vi "TestReadWrite.vi"() -> ()   [LabVIEW 2017, in "JKI Simple Localization.lvlib"]
uses:
  API/JKI Simple Localization.lvlib
panel:
  out "error out":errorcluster
  in  "Dictionary File Path":path
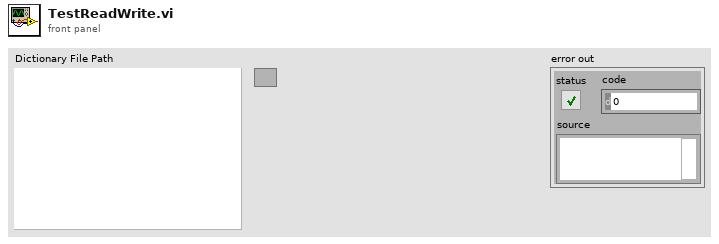
[diagram p1: front panel]
types:
  T1 = typedef "JKI Simple Localization.lvlib/Dictionary--Cluster.ctl" = cluster{"Languages":string[], "Fonts":T2[], "Phrase Dictionary":T3[]}
  T2 = typedef "JKI Simple Localization.lvlib/FontCluster.ctl" = cluster{"Language":string, "Name":string, "Color":u32}
  T3 = typedef "JKI Simple Localization.lvlib/Phrase Dictionary.ctl" = cluster{"Key":string, "Phrases":string[]}
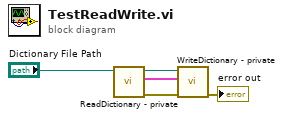
[diagram p0: block diagram]
diagram:
  n1 = call "ReadDictionary - private.vi"("Dictionary File Path"="Dictionary File Path") -> ("error out"=w3:errorcluster, "Dictionary"=w4:T1, "Dictionary File Path out"=w5:path)  [unwired: 8 in]
  n2 = call "WriteDictionary - private.vi"("error in (no error)"=w3, "Localization"=w4, "Dictionary Path"=w5) -> ("error out"=→"error out":errorcluster)  [unwired: 7 in, 1 out]
